vi "Control Panel.vi"(8 "error in (no error)":errorcluster, 11 "LCD Retarder in":refnum<class "LCD Retarder.lvclass">) -> (0 "error out":errorcluster, 3 "LCD Retarder out":refnum<class "LCD Retarder.lvclass">)   [LabVIEW 2009, in "LCD Retarder.lvclass"]
uses:
  LCD Retarder.lvclass
  Utility Classes/Readable/Readable.lvclass
  LCD Retarder.lvclass/LCD Retarder.ctl
  Main/Global/Flags.vi
panel:
  in  "How many periods?":i32=1 min=1 max=50 step=1
  out "Current Retardance":dbl[unit]
  in  "Frequency":dbl
  in  "Retardance 2":dbl
  in  "Retardance 1":dbl
  in  "Alternate":bool
  in  "stop":bool
  out "error":bool caption="Error"
  in  "Check for Instrument":bool
  out "Current Retardance":dbl[unit] caption="Retardance"
  out "Ready":bool
  in  "waveoptions":T1(radio) caption="Wave Options"
  in  "Wavelength":dbl[unit]=7.81e-07
  out "Title":string="LCD Retarder Control Program"
  in  "Zero":bool
  in  "Set\nRetardance":bool
  in  "Goto Retardance":dbl[unit]
  in  "Exit":bool
  # "between"
  # "and"
  # "at"
  # "Hz"
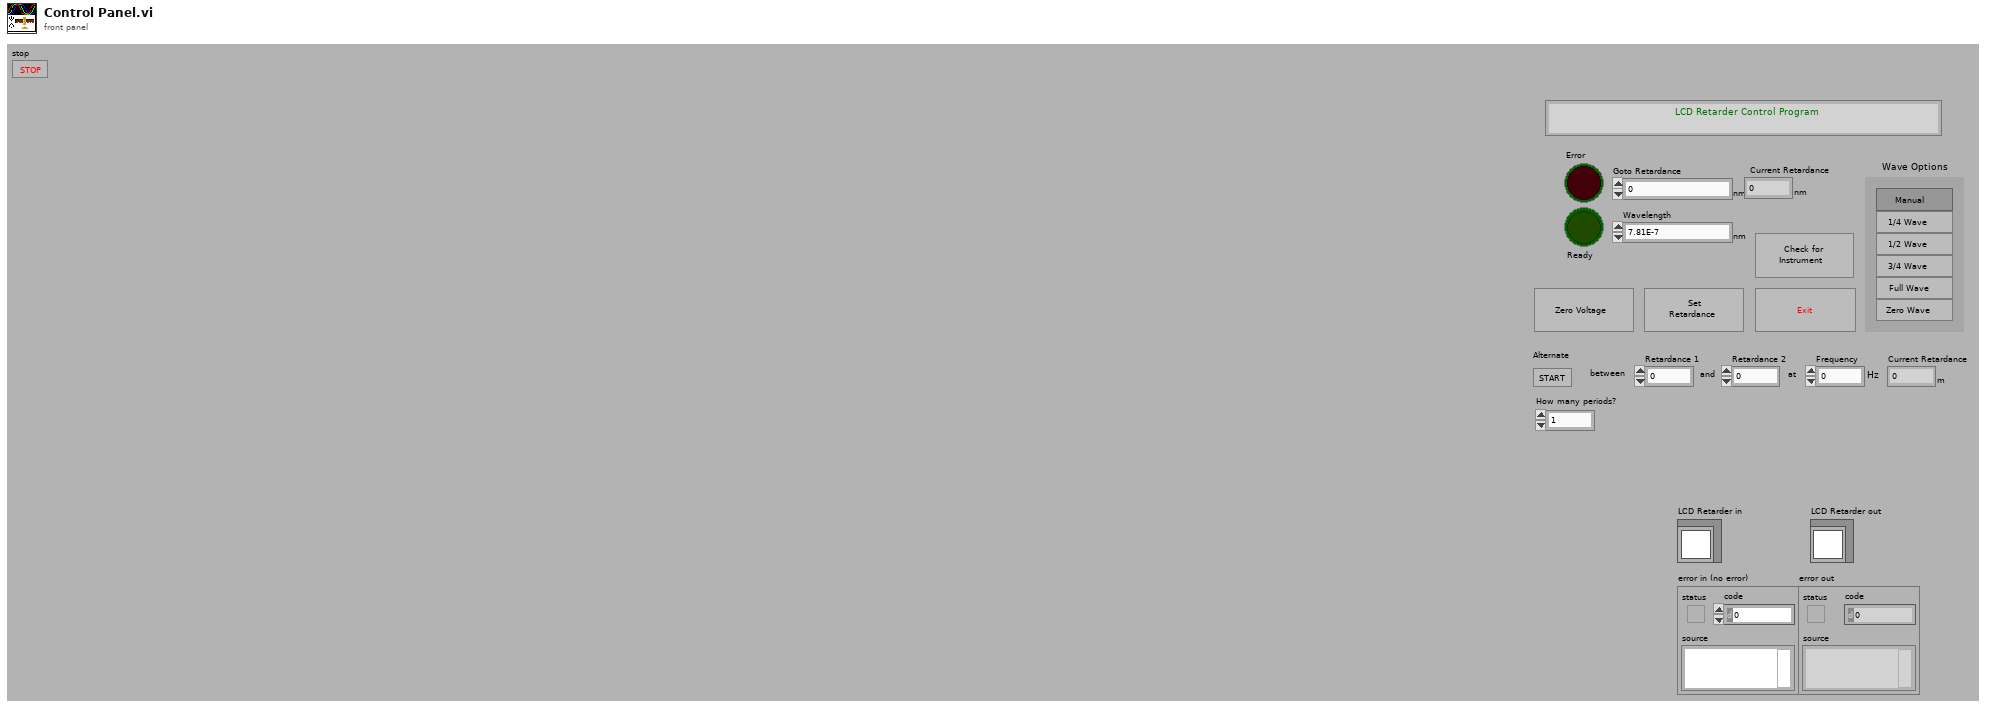
[diagram p1: front panel]
types:
  T1 = enum32{"Manual", "1/4 Wave", "1/2 Wave", "3/4 Wave", "Full Wave", "Zero Wave"}
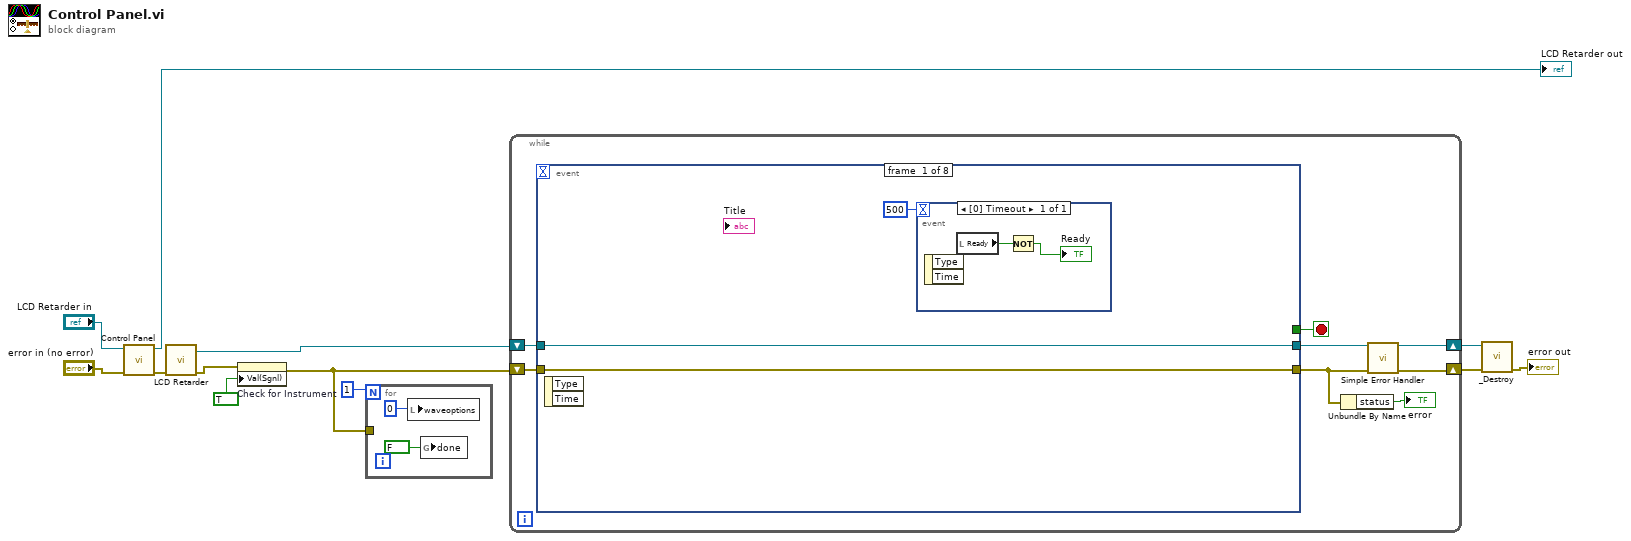
[diagram p0: block diagram]
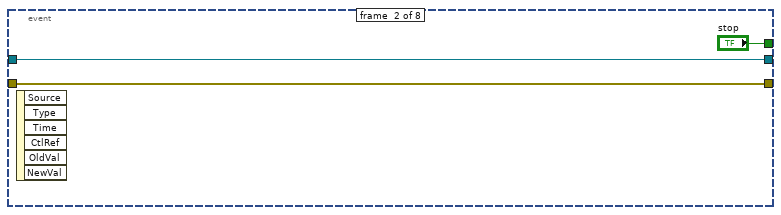
[diagram p2: hidden frame]
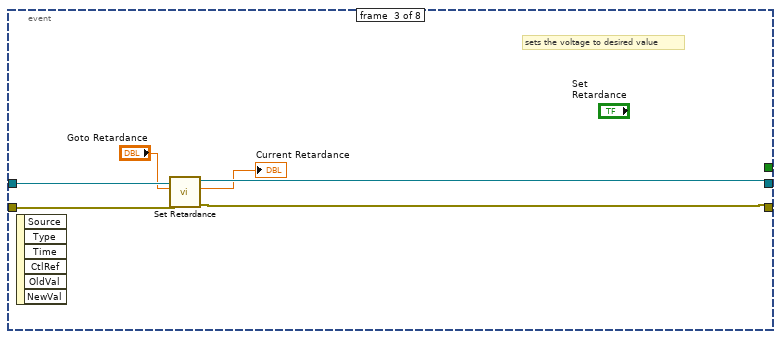
[diagram p3: hidden frame]
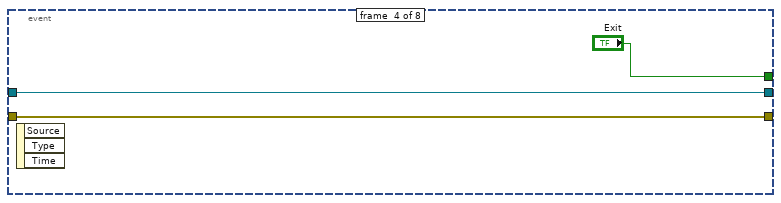
[diagram p4: hidden frame]
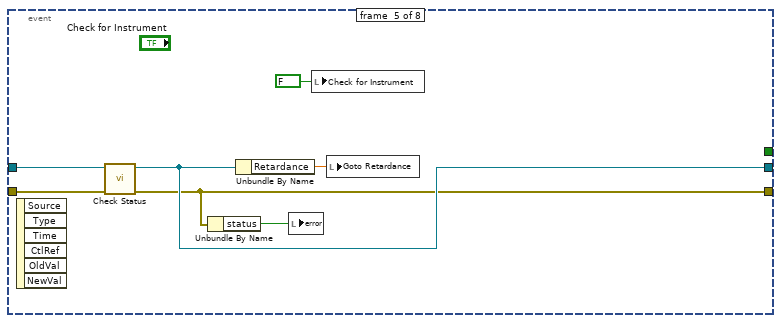
[diagram p5: hidden frame]
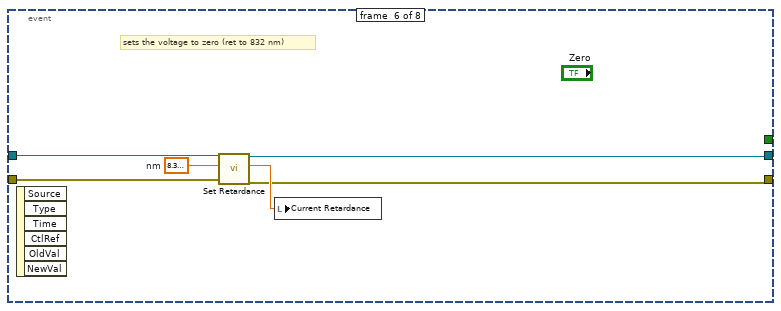
[diagram p6: hidden frame]
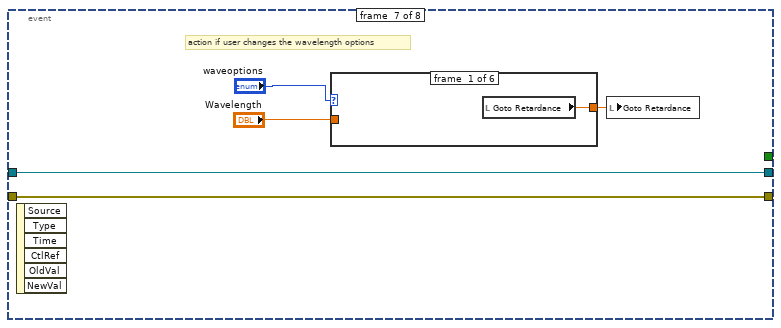
[diagram p7: hidden frame]
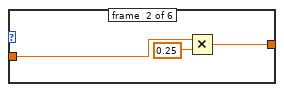
[diagram p8: hidden frame]
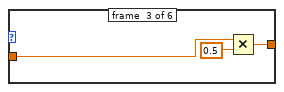
[diagram p9: hidden frame]
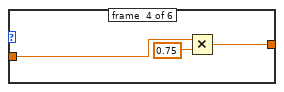
[diagram p10: hidden frame]
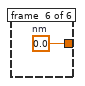
[diagram p12: hidden frame]
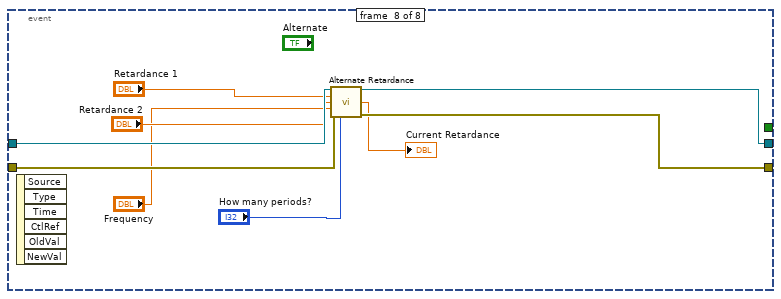
[diagram p13: hidden frame]
diagram:
  n1 = call-parent "Control Panel.vi"("error in (no error)"="error in (no error)", "Instrument in"="LCD Retarder in") -> ("error out"=w12:errorcluster, "Instrument out"=→"LCD Retarder out":refnum<class "LCD Retarder.lvclass">)  [unwired: 8 out]
  n2 = call "LCD Retarder.vi"("error in"=w12) -> ("errorOUT"=w4:errorcluster, "LCD out"=w1:refnum<class "LCD Retarder.lvclass">)  [unwired: 2 in, 7 out]
  n3 = property on="Check for Instrument" class="Bool (strict)"(error in=w4, "Val(Sgnl)"=TRUE ("Value (Signaling)")) -> (error out=w3:errorcluster)  [unwired: 1 in, 1 out]
  n4 = for {
    N: 1 -> [_]
    tunnel: w3 -> [_]
    n5 = local write "waveoptions"(0) -> ()
    n6 = global write "Flags.vi" "done"(FALSE) -> ()
  }
  n7 = while {
    shift-right: [w19] -> w11
    shift-left: w1 -> [w18]
    shift-right: [w16] -> w10
    shift-left: w3 -> [w20]
    stop <- w21 stop-if-true
    n8 = event shown="[7] \"Alternate\": Value Change" {
      selector: _ -> [_ _ _ _ _ _ _ _]
      dyn-events: _ -> [_ _ _ _ _ _ _ _]
      timeout: _ -> [_ _ _ _ _ _ _ _]
      tunnel: [_ "stop" _ "Exit" _ _ _ _] -> w21
      tunnel: [w23 w28 w34 w37 w40 w47 w54 w75] -> w17
      tunnel: w20 -> [w23 w28 w32 w37 w45 w48 w54 w76]
      tunnel: [w24 w27 w35 w38 w42 w46 w55 w74] -> w19
      tunnel: w18 -> [w24 w27 w33 w38 w44 w49 w55 w77]
      event #0 {
        n9 = event-data() -> ()  [unwired: 3 out]
        n10 = event shown="[0] Timeout" {
          selector: _ -> [_]
          dyn-events: _ -> [_]
          timeout: 500 -> [_]
          event [0] Timeout {
            n11 = event-data() -> ()  [unwired: 1 in, 2 out]
            n12 = local read "Ready"() -> (w26:bool)
            n13 = Not(x=w26) -> (.not. x?=→"Ready":bool)
          }
        }
      }
      event #1 {
        n14 = event-data() -> ()  [unwired: 7 out]
      }
      event #2 {
        # "sets the voltage to desired value"
        n15 = event-data() -> ()  [unwired: 7 out]
        n16 = call "Set Retardance.vi"("errorIN"=w32, "Retardance"="Goto Retardance", "LCD in"=w33) -> ("errorOUT"=w34:errorcluster, "Retardance out"=→"Current Retardance":dbl[unit], "LCD out"=w35:refnum<class "LCD Retarder.lvclass">)  [unwired: 6 out]
      }
      event #3 {
        n17 = event-data() -> ()  [unwired: 4 out]
      }
      event #4 {
        n18 = event-data() -> ()  [unwired: 7 out]
        n19 = call-dynamic "Check Status.vi"("error in (no error)"=w45, "LCD Retarder in"=w44) -> ("error out"=w40:errorcluster, "LCD Retarder out"=w42:refnum<class "LCD Retarder.lvclass">)  [unwired: 8 out]
        n20 = Unbundle By Name(w40) -> ("status"=w39:bool)
        n21 = Unbundle By Name(w42) -> ("Retardance"=w43:dbl[unit])
        n22 = local write "error"(w39) -> ()
        n23 = local write "Check for Instrument"(FALSE ("Check for Instrument")) -> ()
        n24 = local write "Goto Retardance"(w43) -> ()
      }
      event #5 {
        w50 = dbl[unit] 8.32e-07  # nm
        # "sets the voltage to zero (ret to 832 nm)"
        n25 = event-data() -> ()  [unwired: 7 out]
        n26 = call "Set Retardance.vi"("errorIN"=w48, "Retardance"=w50, "LCD in"=w49) -> ("errorOUT"=w47:errorcluster, "Retardance out"=w51:dbl[unit], "LCD out"=w46:refnum<class "LCD Retarder.lvclass">)  [unwired: 6 out]
        n27 = local write "Current Retardance"(w51) -> ()
      }
      event #6 {
        # "action if user changes the wavelength options"
        n28 = event-data() -> ()  [unwired: 7 out]
        n29 = case shown="\"1/4 Wave\"" "waveoptions" {
          tunnel: "Wavelength" -> [_ w60 w63 w66 w67 _]
          tunnel: [w57 w58 w61 w64 w67 w68] -> w56
          frame #0 {
            n30 = local read "Goto Retardance"() -> (w57:dbl[unit])
          }
          frame #1 {
            n31 = Multiply(x=w60, y=0.25) -> (x*y=w58:dbl[unit])
          }
          frame #2 {
            n32 = Multiply(x=w63, y=0.5) -> (x*y=w61:dbl[unit])
          }
          frame #3 {
            n33 = Multiply(x=w66, y=0.75) -> (x*y=w64:dbl[unit])
          }
          frame #4 {
          }
          frame #5 {
            w68 = dbl[unit] 0.0  # nm
          }
        }
        n34 = local write "Goto Retardance"(w56) -> ()
      }
      event #7 {
        n35 = event-data() -> ()  [unwired: 7 out]
        n36 = call "Alternate Retardance.vi"("LCD Retarder in"=w77, "Retardance 1"="Retardance 1", "Retardance 2"="Retardance 2", "Frequency"="Frequency", "error in (no error)"=w76, "Cycles"="How many periods?") -> ("LCD Retarder out"=w74:refnum<class "LCD Retarder.lvclass">, "Current Retardance"=→"Current Retardance":dbl[unit], "error out"=w75:errorcluster)  [unwired: 7 in]
      }
    }
    n37 = Unbundle By Name(w17) -> ("status"=→"error":bool)
    n38 = call <vilib>:"Simple Error Handler.vi"("error in (no error)"=w17) -> ("error out"=w16:errorcluster)  [unwired: 1 in, 7 out]
  }
  n39 = call-dynamic "_Destroy.vi"("error in (no error)"=w10, "LCD Retarder in"=w11) -> ("error out"=→"error out":errorcluster)  [unwired: 9 out]
